vi "determine_range_line.vi"(6 "Data":sgl[][](array[numeric]), 8 "Y vector":sgl[](array[numeric]), 9 "X vector":sgl[](array[numeric])) -> (1 "Use X/Y vectors?":bool=TRUE, 3 "Data Dimension":cluster{"X":i32, "Y":i32})   [LabVIEW 2020]
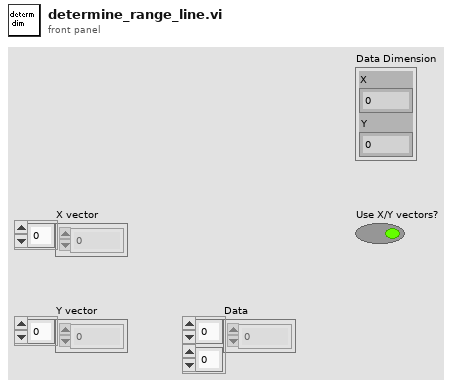
[diagram p1: front panel]
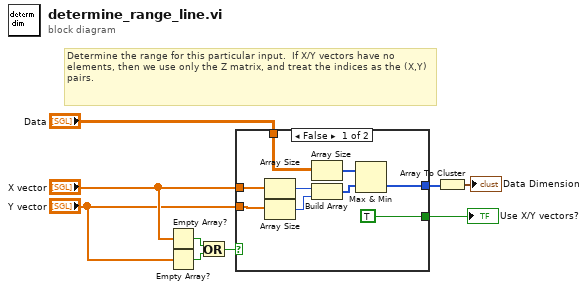
[diagram p0: block diagram]
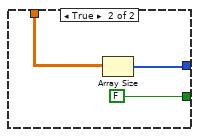
[diagram p2: hidden frame]
diagram:
  # "Determine the range for this particular input.  If X/Y vectors have no elements, then we use only the Z matrix, and treat the indices as the (X,Y) pairs."
  n1 = Empty Array?(array="X vector") -> (empty?=w9:bool)
  n2 = Empty Array?(array="Y vector") -> (empty?=w8:bool)
  n3 = Or(x=w9, y=w8) -> (x .or. y?=w7:bool)
  n4 = case shown="False" w7 {
    tunnel: "Data" -> [w18 w21]
    tunnel: [w13 w20] -> w5
    tunnel: "X vector" -> [w11 _]
    tunnel: "Y vector" -> [w10 _]
    tunnel: [TRUE FALSE] -> w1
    frame False {
      n5 = Array Size(array=w11) -> (size(s)=w16:i32)
      n6 = Array Size(array=w10) -> (size(s)=w15:i32)
      n7 = Array Size(array=w18) -> (size(s)=w17:i32[])
      n8 = Build Array(w16, w15) -> (w14:i32[])
      n9 = Max & Min(x=w17, y=w14) -> (min(x,y)=w13:i32[])  [unwired: 1 out]
    }
    frame True {
      n10 = Array Size(array=w21) -> (size(s)=w20:i32[])
    }
  }
  "Use X/Y vectors?" <- w1
  n11 = Array To Cluster(array=w5) -> (cluster=→"Data Dimension":cluster{"[0]":i32, "[1]":i32})
